vi "DriveSet6(SubVI).vi"(9 "Left":dbl format="%#_13g", 10 "Right":dbl format="%#_13g", 11 "output cluster":T1) -> ()   [LabVIEW 2017]
uses:
  FRC SimulatedRSC/DriveMotors.ctl
  <vilib>/Rock Robotics/WPI/MotorControl/WPI_MotorControlDeviceRef.ctl
  <vilib>/Rock Robotics/WPI/MotorControl/WPI_MotorControlType.ctl
  <vilib>/Rock Robotics/SystemInterfaces/DIO/FPGA_DIOPWMChannel.ctl
  <vilib>/Rock Robotics/WPI/PWM/WPI_PWMDeadband.ctl
  <vilib>/Rock Robotics/SystemInterfaces/DIO/FPGA_DIOChannel.ctl
  <vilib>/Rock Robotics/WPI/ThirdParty/Phoenix-LabVIEW/Motor Controller/Controls/CTRE_Phoenix_MotorControl_ControlMode.ctl
  <vilib>/Rock Robotics/WPI/ThirdParty/Phoenix-LabVIEW/Motor Controller/Get/CTRE_Phoenix_MotorController_GetSelectedSensorData.vi
  <vilib>/Rock Robotics/Network Tables/NT Read Number.vi
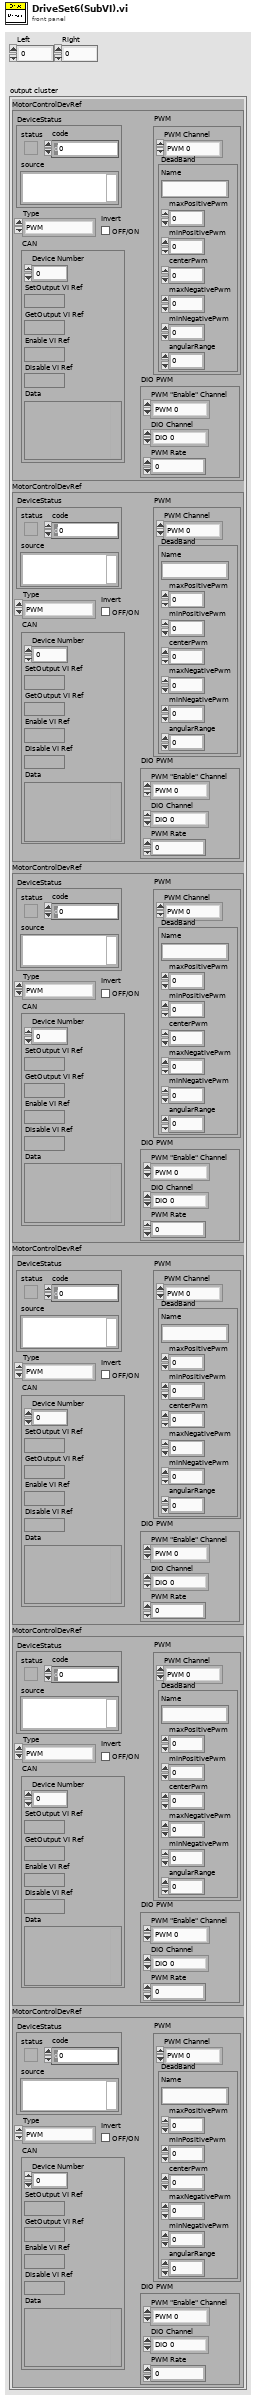
[diagram p1: front panel]
types:
  T1 = typedef "DriveMotors.ctl" = cluster{"MotorControlDevRef":T2, "MotorControlDevRef":T2, "MotorControlDevRef":T2, "MotorControlDevRef":T2, "MotorControlDevRef":T2, "MotorControlDevRef":T2}
  T2 = typedef "WPI_MotorControlDeviceRef.ctl" = cluster{"DeviceStatus":errorcluster, "Type":T3, "PWM":cluster{"PWM Channel":T4, "DeadBand":T5}, "CAN":cluster{"Device Number":u8, "SetOutput VI Ref":variant, "GetOutput VI Ref":variant, "Enable VI Ref":variant, "Disable VI Ref":variant, "Data":variant}, "Invert":bool, "DIO PWM":cluster{"PWM \"Enable\" Channel":T4, "DIOChannel":T6, "PWM Rate":dbl}}
  T3 = typedef "WPI_MotorControlType.ctl" = enum16{"PWM", "CAN", "DIO PWM"}
  T4 = typedef "FPGA_DIOPWMChannel.ctl" = enum8{"PWM 0", "PWM 1", "PWM 2", "PWM 3", "PWM 4", "PWM 5", "PWM 6", "PWM 7", "PWM 8", "PWM 9", "PWM MXP 0", "PWM MXP 1", "PWM MXP 2", "PWM MXP 3", "PWM MXP 4", "PWM MXP 5", "PWM MXP 6", "PWM MXP 7", "PWM MXP 8", "PWM MXP 9", "Invalid"}
  T5 = typedef "WPI_PWMDeadband.ctl" = cluster{"Name":string, "maxPositivePwm":i32, "minPositivePwm":i32, "centerPwm":i32, "maxNegativePwm":i32, "minNegativePwm":i32, "angularRange":u16}
  T6 = typedef "FPGA_DIOChannel.ctl" = enum8{"DIO 0", "DIO 1", "DIO 2", "DIO 3", "DIO 4", "DIO 5", "DIO 6", "DIO 7", "DIO 8", "DIO 9", "DIO MXP 0", "DIO MXP 1", "DIO MXP 2", "DIO MXP 3", "DIO MXP 4", "DIO MXP 5", "DIO MXP 6", "DIO MXP 7", "DIO MXP 8", "DIO MXP 9", "DIO MXP 10", "DIO MXP 11", "DIO MXP 12", "DIO MXP 13", "DIO MXP 14", "DIO MXP 15", "SPI Port CS1", "SPI Port CS2", "SPI Port CS3", "SPI Port MISO", "SPI Port MOSI", "Invalid"}
  T7 = typedef "CTRE_Phoenix_MotorControl_ControlMode.ctl" = u16
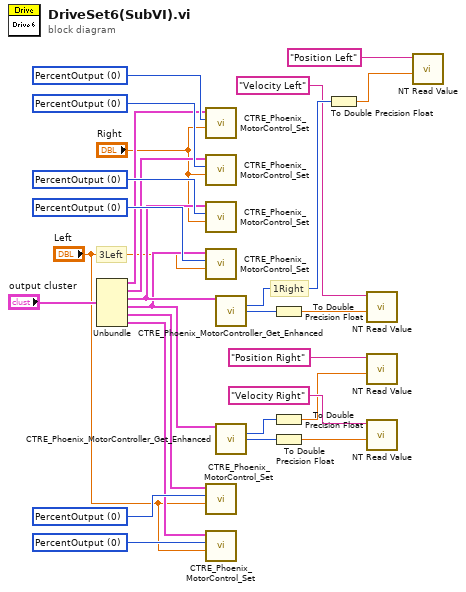
[diagram p0: block diagram]
diagram:
  w4 = T7 0 items=["PercentOutput"=0, "Position"=1, "Velocity"=2, "Current"=3, "Follower"=5, "MotionProfile"=6, "MotionMagic"=7, "MotionMagicArc"=8, "MotionProfileArc"=10, "Disabled"=15] ("Control Mode")
  w5 = T7 0 items=["PercentOutput"=0, "Position"=1, "Velocity"=2, "Current"=3, "Follower"=5, "MotionProfile"=6, "MotionMagic"=7, "MotionMagicArc"=8, "MotionProfileArc"=10, "Disabled"=15] ("Control Mode")
  w9 = T7 0 items=["PercentOutput"=0, "Position"=1, "Velocity"=2, "Current"=3, "Follower"=5, "MotionProfile"=6, "MotionMagic"=7, "MotionMagicArc"=8, "MotionProfileArc"=10, "Disabled"=15] ("Control Mode")
  w10 = T7 0 items=["PercentOutput"=0, "Position"=1, "Velocity"=2, "Current"=3, "Follower"=5, "MotionProfile"=6, "MotionMagic"=7, "MotionMagicArc"=8, "MotionProfileArc"=10, "Disabled"=15] ("Control Mode")
  w25 = T7 0 items=["PercentOutput"=0, "Position"=1, "Velocity"=2, "Current"=3, "Follower"=5, "MotionProfile"=6, "MotionMagic"=7, "MotionMagicArc"=8, "MotionProfileArc"=10, "Disabled"=15] ("Control Mode")
  w26 = T7 0 items=["PercentOutput"=0, "Position"=1, "Velocity"=2, "Current"=3, "Follower"=5, "MotionProfile"=6, "MotionMagic"=7, "MotionMagicArc"=8, "MotionProfileArc"=10, "Disabled"=15] ("Control Mode")
  # "3Left"
  # "1Right"
  n1 = Unbundle("output cluster") -> ("MotorControlDevRef"=w8:T2, "MotorControlDevRef"=w7:T2, "MotorControlDevRef"=w12:T2, "MotorControlDevRef"=w11:T2, "MotorControlDevRef"=w6:T2, "MotorControlDevRef"=w3:T2)
  n2 = call <vilib>:"CTRE_Phoenix_MotorControl_Set.vi"("Output"="Right", "Control Mode"=w10, "PhoenixMotorControlDevRef"=w8) -> ()  [unwired: 7 in, 2 out]
  n3 = call <vilib>:"CTRE_Phoenix_MotorControl_Set.vi"("Output"="Right", "Control Mode"=w9, "PhoenixMotorControlDevRef"=w7) -> ()  [unwired: 7 in, 2 out]
  n4 = call <vilib>:"CTRE_Phoenix_MotorControl_Set.vi"("Output"="Right", "Control Mode"=w25, "PhoenixMotorControlDevRef"=w12) -> ()  [unwired: 7 in, 2 out]
  n5 = call <vilib>:"CTRE_Phoenix_MotorControl_Set.vi"("Output"="Left", "Control Mode"=w26, "PhoenixMotorControlDevRef"=w11) -> ()  [unwired: 7 in, 2 out]
  n6 = call <vilib>:"CTRE_Phoenix_MotorControl_Set.vi"("Output"="Left", "Control Mode"=w5, "PhoenixMotorControlDevRef"=w6) -> ()  [unwired: 7 in, 2 out]
  n7 = call <vilib>:"CTRE_Phoenix_MotorControl_Set.vi"("Output"="Left", "Control Mode"=w4, "PhoenixMotorControlDevRef"=w3) -> ()  [unwired: 7 in, 2 out]
  n8 = call-poly <vilib>:"CTRE_Phoenix_MotorController_Get_Enhanced.vi"("PhoenixMotorControlDevRef"=w12) -> ("Position (Raw Sensor Units)"=w20:i32, "Velocity (Raw Sensor Units per 100 ms)"=w18:i32)  [unwired: 11 in, 2 out]
  n9 = call-poly <vilib>:"CTRE_Phoenix_MotorController_Get_Enhanced.vi"("PhoenixMotorControlDevRef"=w11) -> ("Position (Raw Sensor Units)"=w24:i32, "Velocity (Raw Sensor Units per 100 ms)"=w22:i32)  [unwired: 11 in, 2 out]
  n10 = To Double Precision Float(number=w18) -> (double precision float=w14:dbl)
  n11 = To Double Precision Float(number=w24) -> (double precision float=w15:dbl)
  n12 = To Double Precision Float(number=w22) -> (double precision float=w13:dbl)
  n13 = To Double Precision Float(number=w20) -> (double precision float=w16:dbl)
  n14 = call-poly <vilib>:"NT Read Value.vi"("Default Value"=w14, "Name"="Velocity Left") -> ()  [unwired: 8 in, 2 out]
  n15 = call-poly <vilib>:"NT Read Value.vi"("Default Value"=w15, "Name"="Position Right") -> ()  [unwired: 8 in, 2 out]
  n16 = call-poly <vilib>:"NT Read Value.vi"("Default Value"=w13, "Name"="Velocity Right") -> ()  [unwired: 8 in, 2 out]
  n17 = call-poly <vilib>:"NT Read Value.vi"("Default Value"=w16, "Name"="Position Left") -> ()  [unwired: 8 in, 2 out]
